vi "Zmienn_globalne.vi"() -> ()   [LabVIEW 2023]
panel:
  in  "Woda z wodociagu":bool
  in  "Awaryjne wylaczenie":bool
  out "Brak wody w zbiorniku i wodociagu":bool
  out "Brak wody w zbiorniku":bool
  out "Zepsuty zraszacz":bool
  out "Niedzialajacy czujnik wilgotnosci":bool
  out "Niedzialajacy czujnik temperatury":bool
  in  "Poziom wody w zbiorniku":string
  out "Niski poziom zbiornika":bool
  in  "Aktualne przyspieszenie czas":dbl
  in  "Wilgotnosc":dbl(slide)=50.0 scale=0.0..100.0
  in  "Naslonecznienie":dbl(slide)=50.0 scale=0.0..100.0
  in  "Rok":i32
  in  "Miesiac":i32
  in  "Dzien":i32
  in  "Godziny":i32
  in  "Minuty":i32
  in  "Oproznianie wody":dbl
  in  "Aktualny stan napelnienia":dbl=50.0
  in  "Opady deszczu":dbl
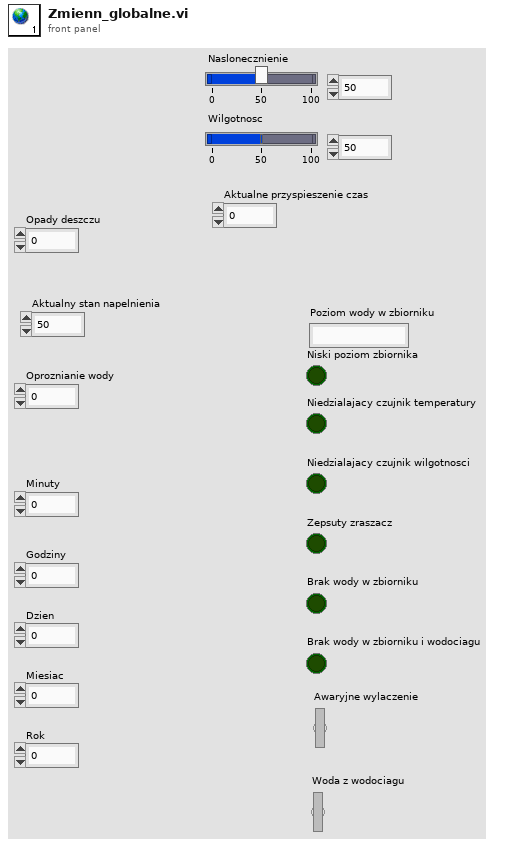
[diagram p1: front panel]
diagram:
